vi "Read Interpolation File.vi"(8 "error in":errorcluster, 10 "file path (dialog if empty)":path) -> (0 "error out":errorcluster, 1 "Profiles []":cluster{"Profile":dbl[][]}[](array[cluster]), 2 "Profiles":string[](array[string]), 3 "Raw Data":string[][](array[string]), 4 "xName":string, 5 "xUnit":string, 6 "yName":string, 7 "yUnit":string)   [LabVIEW 2019, in "Profile Interpolation Shared.lvlib"]
uses:
  469b4b88-89ce-43a1-bf6f-93cb86ea8270.vi
  <vilib>/Utility/file.llb/Read Delimited Spreadsheet (string).vi
  <userlib>/_OpenG.lib/array/array.llb/Filter 1D Array with Scalar (String)__ogtk.vi
  Profile Interpolation Shared.lvlib
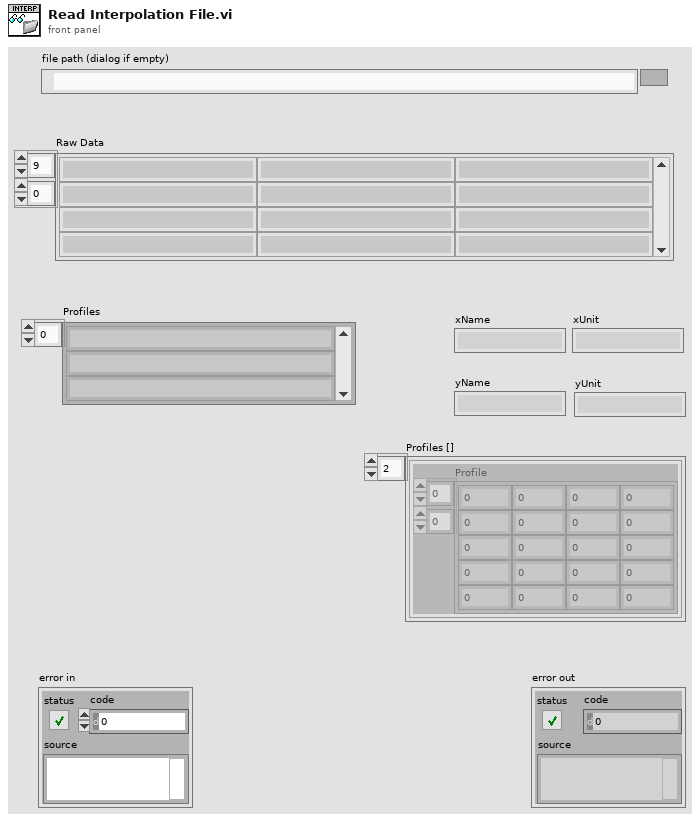
[diagram p1: front panel]
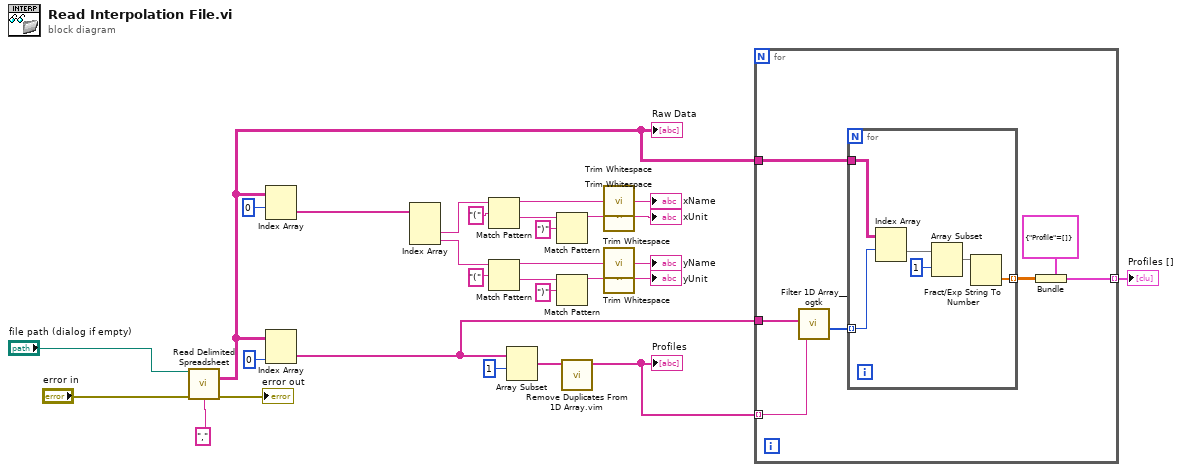
[diagram p0: block diagram]
diagram:
  n1 = call-poly <vilib>:"Read Delimited Spreadsheet.vi"("file path (dialog if empty)"="file path (dialog if empty)", "error in (no error)"="error in", "delimiter (\\t)"="," ("delimiter (\\t)")) -> ("all rows"=w3:string[][], "error out"=→"error out":errorcluster)  [unwired: 7 in, 4 out]
  "Raw Data" <- w3
  n2 = Index Array(array=w3, index (row)=0) -> (element=w21:string[])  [unwired: 1 in]
  n3 = Index Array(array=w3, index (col)=0 ("index (row)")) -> (element=w2:string[])  [unwired: 1 in]
  n4 = Index Array(array=w21) -> (element #2=w22:string, element #3=w23:string)  [unwired: 3 in, 1 out]
  n5 = Match Pattern(string=w22, regular expression="(") -> (before substring=w7:string, after substring=w8:string)  [unwired: 1 in, 2 out]
  n6 = Match Pattern(string=w23, regular expression="(") -> (before substring=w13:string, after substring=w14:string)  [unwired: 1 in, 2 out]
  n7 = Array Subset(array=w2, index=1) -> (w20:string[])  [unwired: 1 in]
  n8 = Match Pattern(string=w8, regular expression=")") -> (before substring=w10:string)  [unwired: 1 in, 3 out]
  n9 = Match Pattern(string=w14, regular expression=")") -> (before substring=w16:string)  [unwired: 1 in, 3 out]
  n10 = call "Remove Duplicates From 1D Array.vim"("array"=w20) -> ("array with duplicates removed"=w4:string[])  [unwired: 10 in]
  "Profiles" <- w4
  n11 = call <vilib>:"Trim Whitespace.vi"("string"=w7) -> ("trimmed string"=→"xName":string)  [unwired: 1 in]
  n12 = call <vilib>:"Trim Whitespace.vi"("string"=w10) -> ("trimmed string"=→"xUnit":string)  [unwired: 1 in]
  n13 = call <vilib>:"Trim Whitespace.vi"("string"=w13) -> ("trimmed string"=→"yName":string)  [unwired: 1 in]
  n14 = call <vilib>:"Trim Whitespace.vi"("string"=w16) -> ("trimmed string"=→"yUnit":string)  [unwired: 1 in]
  n15 = for {
    tunnel: w4 -> [w36] mode=indexing
    tunnel: w3 -> [w33]
    tunnel: w2 -> [w35]
    tunnel: [w30] -> w1 mode=indexing
    n16 = call-poly <userlib>:"Filter 1D Array__ogtk.vi"("items to filter"=w36, "array"=w35) -> ("filtered item indices"=w34:i32[])  [unwired: 4 in, 1 out]
    n17 = for {
      tunnel: w34 -> [w41] mode=indexing
      tunnel: w33 -> [w42]
      tunnel: [w40] -> w31 mode=indexing
      n18 = Index Array(array=w42, index (row)=w41) -> (element=w39:string[])  [unwired: 1 in]
      n19 = Array Subset(array=w39, index=1) -> (w37:string[])  [unwired: 1 in]
      n20 = Fract/Exp String To Number(string=w37) -> (number=w40:dbl[])  [unwired: 3 in, 1 out]
    }
    n21 = Bundle(cluster=cluster{"Profile":dbl[][]} {"Profile"=[]} ("Profiles"), "Profile"=w31) -> (w30:cluster{"Profile":dbl[][]})
  }
  "Profiles []" <- w1
